vi "_attribute_write_boolean.vi"(5 "Repeated Capability":string, 7 "Attribute":T1={"Identifier"="", "Descriptive Name"="", "Data Type"=enum."Integer 32", "Command"="", "Access"=enum."Read/Write", "Range Table"="", "Read Callback"="", "Write Callback"="", "Supported Models"="", "Instrument Options"="", "Index"=0, "OPC Wait"=FALSE, "No Status Check"=FALSE, "Cache Only"=FALSE}, 8 "error in":errorcluster caption="error in (no error)", 10 "Boolean in":bool, 11 "VISA resource name":refnum<visa-resource-name>) -> (0 "error out":errorcluster, 3 "VISA resource name out":refnum<visa-resource-name>)   [LabVIEW 2020, in "Rohde&Schwarz RTx Oscilloscopes.lvlib" / "rsidr_core.lvlib"]
uses:
  rsidr_core.lvlib
  type_Attribute.ctl
  type_Attribute_Data_Type.ctl
  type_ReadWriteAccess.ctl
  Rohde&Schwarz RTx Oscilloscopes.lvlib
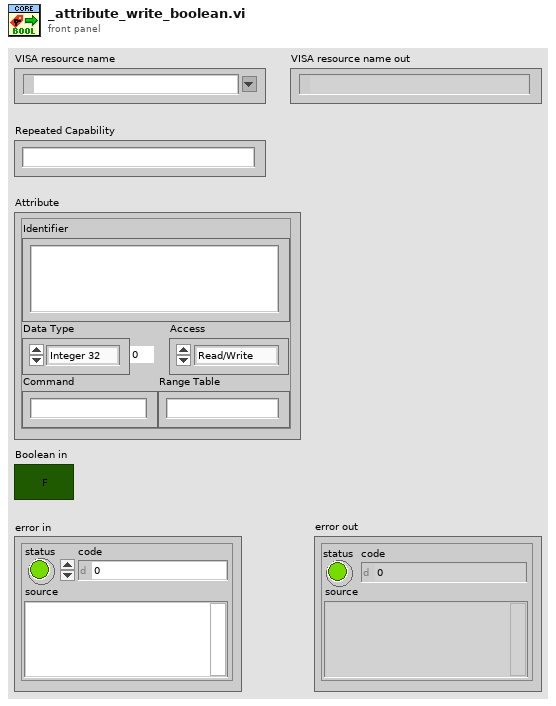
[diagram p1: front panel]
types:
  T1 = typedef "Rohde&Schwarz RTx Oscilloscopes.lvlib/rsidr_core.lvlib/type_Attribute.ctl" = cluster{"Identifier":string, "Descriptive Name":string, "Data Type":T2, "Command":string, "Access":T3, "Range Table":string, "Read Callback":string, "Write Callback":string, "Supported Models":string, "Instrument Options":string, "Index":i32, "OPC Wait":bool, "No Status Check":bool, "Cache Only":bool}
  T2 = typedef "Rohde&Schwarz RTx Oscilloscopes.lvlib/rsidr_core.lvlib/type_Attribute_Data_Type.ctl" = enum16{"Integer 32", "Double", "String", "Boolean", "None", "Integer 64", "RawString"}
  T3 = typedef "Rohde&Schwarz RTx Oscilloscopes.lvlib/rsidr_core.lvlib/type_ReadWriteAccess.ctl" = enum16{"Read Only", "Write Only", "Read/Write"}
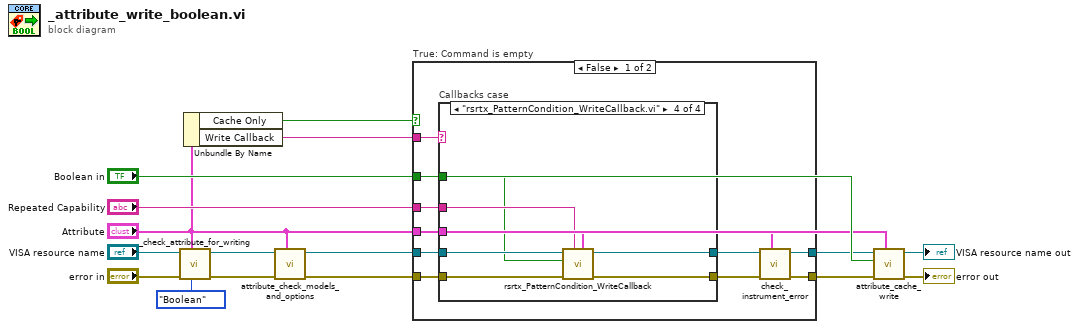
[diagram p0: block diagram]
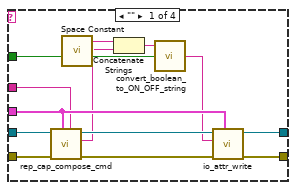
[diagram p2: hidden frame]
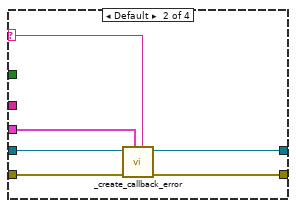
[diagram p3: hidden frame]
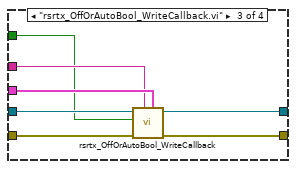
[diagram p4: hidden frame]
diagram:
  n1 = call "_check_attribute_for_writing.vi"("Expected Data Type"=type_Attribute_Data_Type."Boolean" ("Data Type"), "Attribute"="Attribute", "error in"="error in", "VISA resource name"="VISA resource name") -> ("error out"=w8:errorcluster, "VISA resource name out"=w7:refnum<visa-resource-name>)  [unwired: 6 in]
  n2 = Unbundle By Name("Attribute") -> ("Cache Only"=w1:bool, "Write Callback"=w9:string)
  n3 = call "attribute_check_models_and_options.vi"("Attribute"="Attribute", "error in"=w8, "VISA resource name"=w7) -> ("error out"=w6:errorcluster, "VISA resource name out"=w5:refnum<visa-resource-name>)  [unwired: 6 in, 1 out]
  n4 = case "True: Command is empty" shown="False" w1 {
    tunnel: "Repeated Capability" -> [w26 _]
    tunnel: w6 -> [w25 w60]
    tunnel: w5 -> [w24 w61]
    tunnel: "Boolean in" -> [w23 _]
    tunnel: "Attribute" -> [w17 _]
    tunnel: [w18 w61] -> w3
    tunnel: [w19 w60] -> w4
    tunnel: w9 -> [w22 _]
    frame False {
      n5 = case "Callbacks case" shown="\"rsrtx_PatternCondition_WriteCallback.vi\"" w22 {
        selector: w22 -> [_ w40 _ _]
        tunnel: w23 -> [w31 _ w48 w55]
        tunnel: w24 -> [w38 w44 w51 w58]
        tunnel: w25 -> [w36 w45 w52 w59]
        tunnel: w26 -> [w32 _ w49 w56]
        tunnel: [w35 w42 w46 w53] -> w20
        tunnel: [w34 w43 w47 w54] -> w21
        tunnel: w17 -> [w33 w41 w50 w57]
        frame "" {
          n6 = call "rep_cap_compose_cmd.vi"("Repeated Capability"=w32, "Attribute"=w33, "error in"=w36, "VISA resource name"=w38) -> ("error out"=w37:errorcluster, "Command out"=w28:string, "VISA resource name out"=w39:refnum<visa-resource-name>)  [unwired: 5 in]
          n7 = call "Space Constant.vi"() -> ("String"=w27:string)
          n8 = Concatenate Strings(w28, w27) -> (w29:string)
          n9 = call "convert_boolean_to_ON_OFF_string.vi"("boolean value in"=w31, "String to add before (\"\")"=w29) -> ("string value out"=w30:string)  [unwired: 3 in]
          n10 = call "io_attr_write.vi"("Attribute"=w33, "error in"=w37, "write buffer"=w30, "VISA resource name"=w39) -> ("error out"=w34:errorcluster, "VISA resource name out"=w35:refnum<visa-resource-name>)  [unwired: 6 in]
        }
        frame Default {
          n11 = call "_create_callback_error.vi"("Callback Name"=w40, "Attribute"=w41, "error in"=w45, "VISA resource name"=w44) -> ("error out"=w43:errorcluster, "VISA resource name out"=w42:refnum<visa-resource-name>)  [unwired: 6 in]
        }
        frame "rsrtx_OffOrAutoBool_WriteCallback.vi" {
          n12 = call "rsrtx_OffOrAutoBool_WriteCallback.vi"("Attribute"=w50, "Repeated Capability"=w49, "error in"=w52, "Attribute Value Boolean"=w48, "VISA resource name"=w51) -> ("error out"=w47:errorcluster, "VISA resource name out"=w46:refnum<visa-resource-name>)  [unwired: 5 in]
        }
        frame "rsrtx_PatternCondition_WriteCallback.vi" {
          n13 = call "rsrtx_PatternCondition_WriteCallback.vi"("Attribute"=w57, "Repeated Capability"=w56, "error in"=w59, "Attribute Value Boolean"=w55, "VISA resource name"=w58) -> ("error out"=w54:errorcluster, "VISA resource name out"=w53:refnum<visa-resource-name>)  [unwired: 5 in]
        }
      }
      n14 = call "check_instrument_error.vi"("Attribute"=w17, "error in"=w21, "VISA resource name"=w20) -> ("error out"=w19:errorcluster, "VISA resource name out"=w18:refnum<visa-resource-name>)  [unwired: 7 in]
    }
    frame True {
    }
  }
  n15 = call "attribute_cache_write.vi"("Attribute"="Attribute", "error in"=w4, "Value in"="Boolean in", "VISA resource name"=w3) -> ("error out"=→"error out":errorcluster, "VISA resource name out"=→"VISA resource name out":refnum<visa-resource-name>)  [unwired: 6 in]
